vi "LAB5.vi"() -> ()   [LabVIEW 2011]
uses:
  <userlib>/KNR LabVIEW Toolkit/Type Definitions/Port Number (for US).ctl
  <userlib>/KNR LabVIEW Toolkit/Type Definitions/Port Number (for DC).ctl
  <userlib>/KNR LabVIEW Toolkit/General/KNR Open (Direct Mode).vi
  <userlib>/KNR LabVIEW Toolkit/DC Motor Control/DC Motor Library.lvlib
  <userlib>/KNR LabVIEW Toolkit/Ultrasonic Control/Ultrasonic Library.lvlib
panel:
  out "right Velocity (cts/sec)":dbl
  out "ultrasonic(cm)":dbl
  out "Ultrasonic output":T1
  in  "Port Number":T2 items=["US1-US4"=0, "US5-US8"=2]
  out "left Velocity (cts/sec)":dbl
  out "Position 2":i32
  out "Position":i32
  in  "Reverse Encoder 2":bool
  in  "Reset Encoder 2":bool
  in  "Reverse Encoder":bool
  in  "Reset Encoder":bool
  in  "Enable Motor":bool
  out "error out":errorcluster
  in  "stop":bool
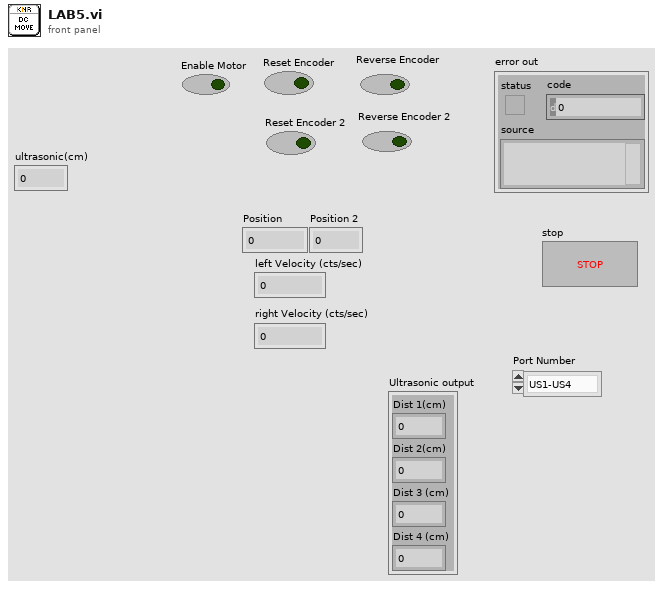
[diagram p1: front panel]
types:
  T1 = cluster{"Dist 1(cm)":dbl, "Dist 2(cm)":dbl, "Dist 3 (cm)":dbl, "Dist 4 (cm)":dbl}
  T2 = typedef "Port Number (for US).ctl" = u16
  T3 = typedef "KNR Reference.ctl" = cluster{"FPGA Session":refnum<class "FPGA Interface Base.lvclass">, "Port Types":T4[]}
  T4 = typedef "Port Type (API).ctl" = enum8{"Unassigned", "DIO", "DC Motor", "RC Motor", "Ultrasonic", "Analog Input"}
  T5 = typedef "Port Number (for DC).ctl" = u16
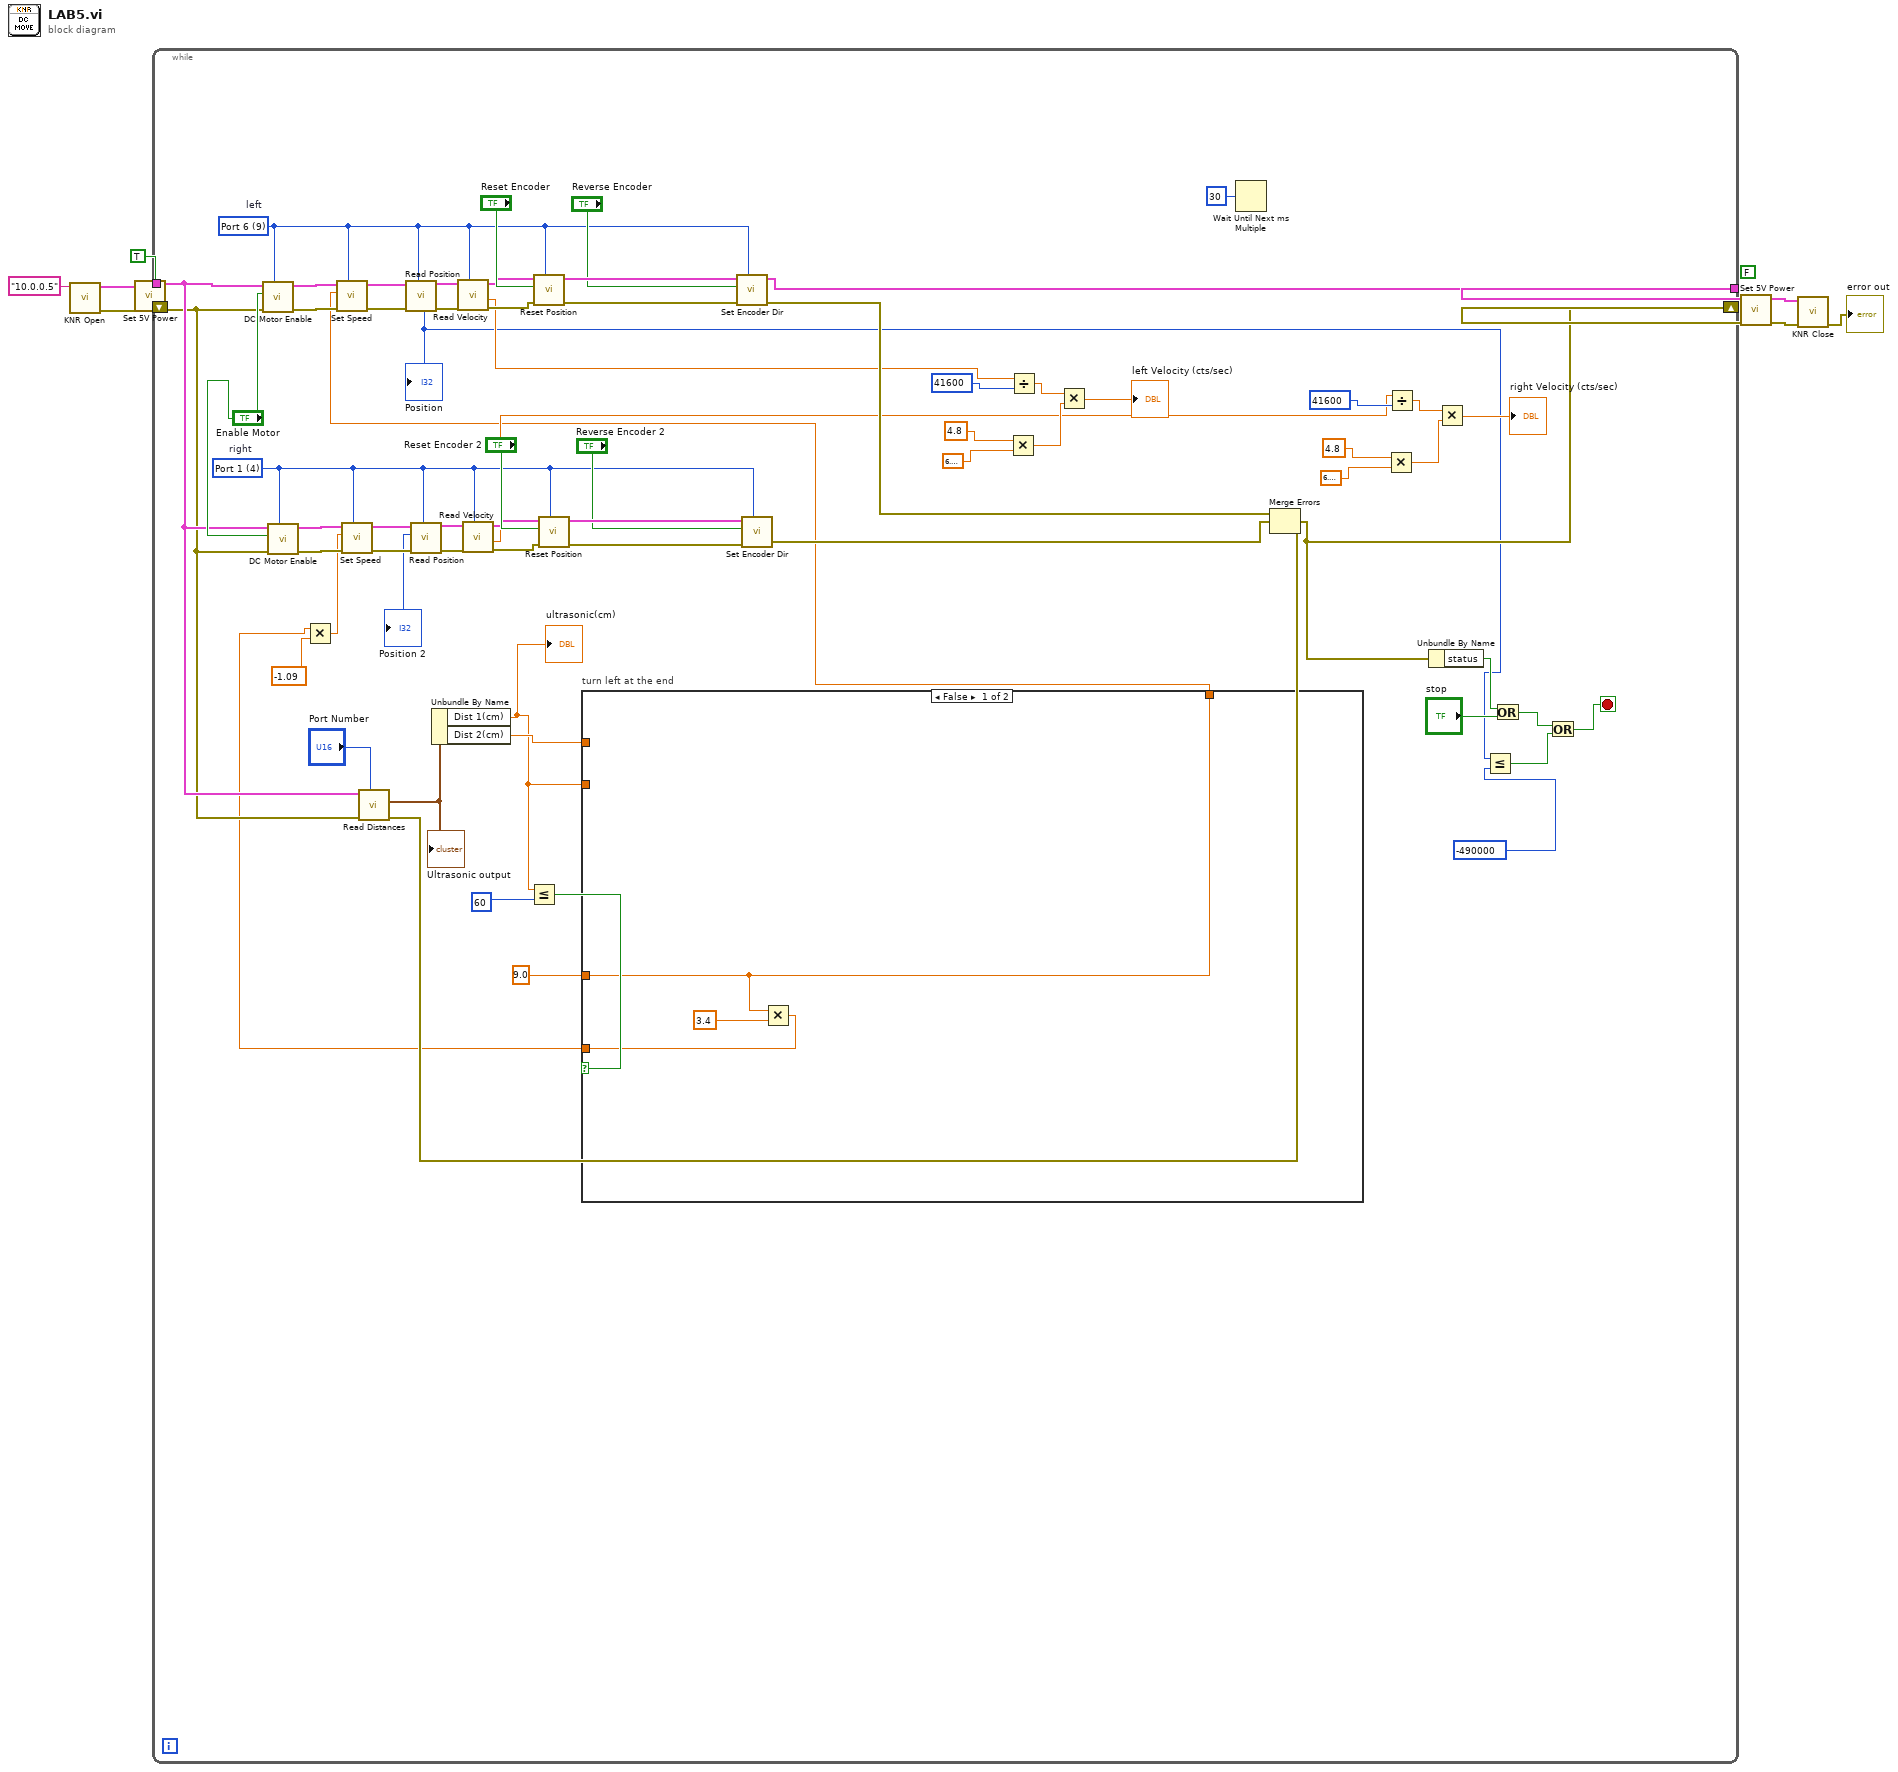
[diagram p0: block diagram]
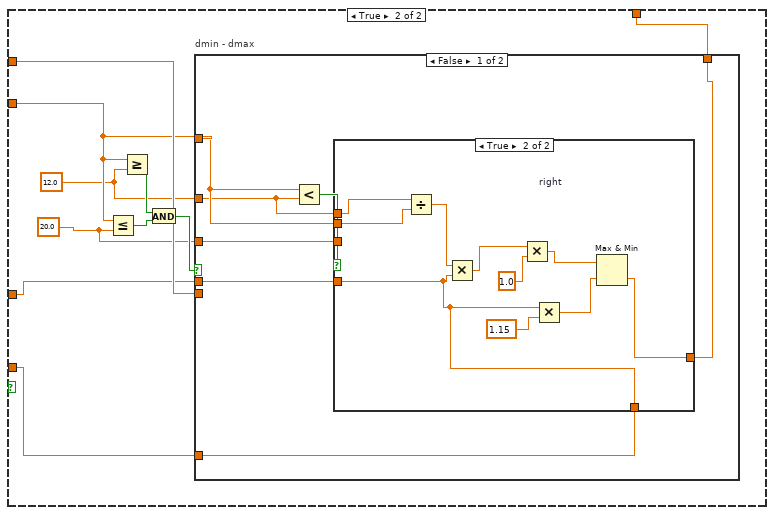
[diagram p2: hidden frame]
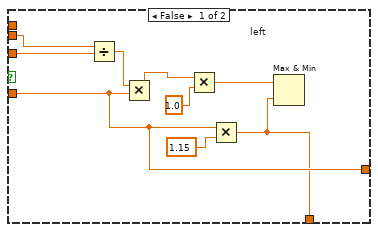
[diagram p3: hidden frame]
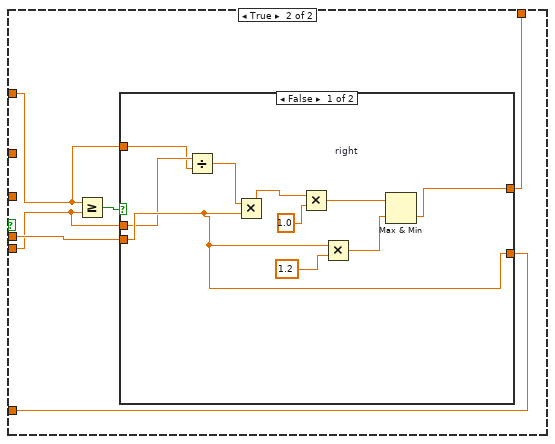
[diagram p4: hidden frame]
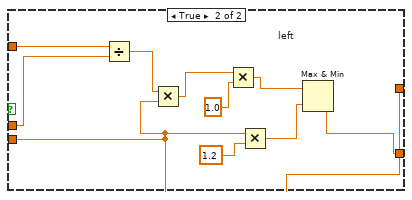
[diagram p5: hidden frame]
diagram:
  (unwired) FALSE ("5V Power")
  n1 = call-poly <userlib>:"KNR Open.vi"("IP Address (Default: 10.0.0.5)"="10.0.0.5") -> ("error out"=w10:errorcluster, "KNR Out"=w11:T3)  [unwired: 9 in]
  n2 = call <userlib>:"Set 5V Power.vi"("error in (no error)"=w10, "5V Power"=TRUE, "KNR In"=w11) -> ("error out"=w7:errorcluster, "KNR Out"=w8:T3)  [unwired: 7 in]
  n3 = while {
    tunnel: w8 -> [w21]
    shift-right: [w46] -> w2
    shift-left: w7 -> [w20]
    tunnel: [w51] -> w1
    stop <- w23 stop-if-true
    w59 = T5 4 items=["Port 1"=4, "Port 2"=5, "Port 3"=6, "Port 4"=7, "Port 5"=8, "Port 6"=9, "Port 7"=10]  # right
    w72 = T5 9 items=["Port 1"=4, "Port 2"=5, "Port 3"=6, "Port 4"=7, "Port 5"=8, "Port 6"=9, "Port 7"=10]  # left
    n4 = call <userlib>:"DC Motor Enable.vi"("Port Number"=w72, "error in (no error)"=w20, "Enable Motor"="Enable Motor", "KNR In"=w21) -> ("error out"=w73:errorcluster, "KNR Out"=w74:T3)  [unwired: 6 in]
    n5 = call <userlib>:"DC Motor Enable.vi"("Port Number"=w59, "error in (no error)"=w20, "Enable Motor"="Enable Motor", "KNR In"=w21) -> ("error out"=w60:errorcluster, "KNR Out"=w61:T3)  [unwired: 6 in]
    n6 = call <userlib>:"Read Distances.vi"("Port Number"="Port Number", "error in (no error)"=w20, "KNR In"=w21) -> ("error out"=w43:errorcluster, "Ultrasonic output"=w44:T1)  [unwired: 6 in, 1 out]
    "Ultrasonic output" <- w44
    n7 = Unbundle By Name(w44) -> ("Dist 1(cm)"=w17:dbl, "Dist 2(cm)"=w18:dbl)
    "ultrasonic(cm)" <- w17
    n8 = Less Or Equal?(x=w17, y=60) -> (x <= y?=w25:bool)
    n9 = case "turn left at the end" shown="False" w25 {
      tunnel: w17 -> [_ w88]
      tunnel: [w82 w90] -> w16
      tunnel: [w80 w89] -> w15
      tunnel: 9.0 ("V") -> [w82 w91]
      tunnel: w18 -> [_ w92]
      frame False {
        n10 = Multiply(x=w82, y=3.4) -> (x*y=w80:dbl)
      }
      frame True {
        w83 = 20.0 ("D max")
        w84 = 12.0 ("D max")
        n11 = Less Or Equal?(x=w88, y=w83) -> (x <= y?=w86:bool)
        n12 = Greater Or Equal?(x=w88, y=w84) -> (x >= y?=w87:bool)
        n13 = And(x=w87, y=w86) -> (x .and. y?=w85:bool)
        n14 = case "dmin - dmax" shown="False" w85 {
          tunnel: w88 -> [w98 w123]
          tunnel: w92 -> [_ w119]
          tunnel: w84 -> [w95 _]
          tunnel: w91 -> [w97 w122]
          tunnel: [w94 w121] -> w90
          tunnel: [w93 w120] -> w89
          tunnel: w83 -> [w96 _]
          frame False {
            n15 = Less?(x=w98, y=w95) -> (x < y?=w99:bool)
            n16 = case shown="True" w99 {
              tunnel: w98 -> [w101 w109]
              tunnel: w97 -> [w103 w111]
              tunnel: w96 -> [w100 _]
              tunnel: w95 -> [_ w110]
              tunnel: [w103 w112] -> w94
              tunnel: [w102 w111] -> w93
              frame False {
                n17 = Divide(x=w101, y=w100) -> (x/y=w107:dbl)
                n18 = Multiply(x=w107, y=w103) -> (x*y=w106:dbl)
                n19 = Multiply(x=w106, y=1.0) -> (x*y=w104:dbl)
                n20 = Multiply(x=w103, y=1.15) -> (x*y=w102:dbl)
                n21 = Max & Min "left"(x=w104, y=w102) -> ()  [unwired: 2 out]
              }
              frame True {
                n22 = Divide(x=w110, y=w109) -> (x/y=w118:dbl)
                n23 = Multiply(x=w118, y=w111) -> (x*y=w114:dbl)
                n24 = Multiply(x=w114, y=1.0) -> (x*y=w113:dbl)
                n25 = Multiply(x=w111, y=1.15) -> (x*y=w116:dbl)
                n26 = Max & Min "right"(x=w113, y=w116) -> (min(x,y)=w112:dbl)  [unwired: 1 out]
              }
            }
          }
          frame True {
            n27 = Greater Or Equal?(x=w123, y=w119) -> (x >= y?=w124:bool)
            n28 = case shown="False" w124 {
              tunnel: [w131 w137] -> w121
              tunnel: [w127 w135] -> w120
              tunnel: w123 -> [w125 w138]
              tunnel: w122 -> [w127 w137]
              tunnel: w119 -> [w126 w136]
              frame False {
                n29 = Divide(x=w126, y=w125) -> (x/y=w132:dbl)
                n30 = Multiply(x=w132, y=w127) -> (x*y=w130:dbl)
                n31 = Multiply(x=w130, y=1.0) -> (x*y=w128:dbl)
                n32 = Multiply(x=w127, y=1.2) -> (x*y=w134:dbl)
                n33 = Max & Min "right"(x=w128, y=w134) -> (min(x,y)=w131:dbl)  [unwired: 1 out]
              }
              frame True {
                n34 = Divide(x=w138, y=w136) -> (x/y=w144:dbl)
                n35 = Multiply(x=w144, y=w137) -> (x*y=w140:dbl)
                n36 = Multiply(x=w140, y=1.0) -> (x*y=w139:dbl)
                n37 = Multiply(x=w137, y=1.2) -> (x*y=w142:dbl)
                n38 = Max & Min "left"(x=w139, y=w142) -> (min(x,y)=w135:dbl)  [unwired: 1 out]
              }
            }
          }
        }
      }
    }
    n39 = Multiply(x=w15, y=-1.09) -> (x*y=w27:dbl)
    n40 = call <userlib>:"Set Speed.vi"("Port Number"=w72, "error in (no error)"=w73, "Speed (+-100%)"=w16, "KNR In"=w74) -> ("error out"=w70:errorcluster, "KNR Out"=w71:T3)  [unwired: 6 in]
    n41 = call <userlib>:"Set Speed.vi"("Port Number"=w59, "error in (no error)"=w60, "Speed (+-100%)"=w27, "KNR In"=w61) -> ("error out"=w57:errorcluster, "KNR Out"=w58:T3)  [unwired: 6 in]
    n42 = call <userlib>:"Read Position.vi"("Port Number"=w72, "error in (no error)"=w70, "KNR In"=w71) -> ("error out"=w68:errorcluster, "Position"=w12:i32, "KNR Out"=w69:T3)  [unwired: 6 in]
    "Position" <- w12
    n43 = call <userlib>:"Read Position.vi"("Port Number"=w59, "error in (no error)"=w57, "KNR In"=w58) -> ("error out"=w55:errorcluster, "Position"=→"Position 2":i32, "KNR Out"=w56:T3)  [unwired: 6 in]
    n44 = call <userlib>:"Read Velocity.vi"("Port Number"=w72, "error in (no error)"=w68, "KNR In"=w69) -> ("error out"=w66:errorcluster, "Velocity (cts/sec)"=w36:dbl, "KNR Out"=w67:T3)  [unwired: 6 in]
    n45 = call <userlib>:"Read Velocity.vi"("Port Number"=w59, "error in (no error)"=w55, "KNR In"=w56) -> ("error out"=w53:errorcluster, "Velocity (cts/sec)"=w29:dbl, "KNR Out"=w54:T3)  [unwired: 6 in]
    n46 = call <userlib>:"Reset Position.vi"("Port Number"=w72, "error in (no error)"=w66, "Reset"="Reset Encoder", "KNR In"=w67) -> ("error out"=w77:errorcluster, "KNR Out"=w78:T3)  [unwired: 6 in]
    n47 = call <userlib>:"Reset Position.vi"("Port Number"=w59, "error in (no error)"=w53, "Reset"="Reset Encoder 2", "KNR In"=w54) -> ("error out"=w64:errorcluster, "KNR Out"=w65:T3)  [unwired: 6 in]
    n48 = call <userlib>:"Set Encoder Dir.vi"("Port Number"=w72, "error in (no error)"=w77, "Reverse?"="Reverse Encoder", "KNR In"=w78) -> ("error out"=w50:errorcluster, "KNR Out"=w51:T3)  [unwired: 6 in]
    n49 = call <userlib>:"Set Encoder Dir.vi"("Port Number"=w59, "error in (no error)"=w64, "Reverse?"="Reverse Encoder 2", "KNR In"=w65) -> ("error out"=w49:errorcluster)  [unwired: 6 in, 1 out]
    n50 = Multiply(x=4.8, y=6.283185307179586) -> (x*y=w39:dbl)
    n51 = Divide(x=w36, y=41600) -> (x/y=w42:dbl)
    n52 = Multiply(x=w42, y=w39) -> (x*y=→"left Velocity (cts/sec)":dbl)
    n53 = Wait Until Next ms Multiple(millisecond multiple=u32 30) -> ()  [unwired: 1 out]
    n54 = Merge Errors(w50, w49, w43) -> (w46:errorcluster)
    n55 = Multiply(x=4.8, y=6.283185307179586) -> (x*y=w32:dbl)
    n56 = Divide(x=w29, y=41600) -> (x/y=w35:dbl)
    n57 = Unbundle By Name(w46) -> ("status"=w47:bool)
    n58 = Multiply(x=w35, y=w32) -> (x*y=→"right Velocity (cts/sec)":dbl)
    n59 = Less Or Equal?(x=w12, y=-490000) -> (x <= y?=w14:bool)
    n60 = Or(x=w47, y="stop") -> (x .or. y?=w24:bool)
    n61 = Or(x=w24, y=w14) -> (x .or. y?=w23:bool)
  }
  n62 = call <userlib>:"Set 5V Power.vi"("error in (no error)"=w2, "KNR In"=w1) -> ("error out"=w4:errorcluster, "KNR Out"=w5:T3)  [unwired: 8 in]
  n63 = call <userlib>:"KNR Close.vi"("error in (no error)"=w4, "KNR In"=w5) -> ("error out"=→"error out":errorcluster)  [unwired: 9 in]
